vi "SerialUntraOOP.vi"(8 "error in (no error)":errorcluster, 10 "Queue In":T1) -> (0 "error out":errorcluster)   [LabVIEW 2017, in "libVariable.lvlib" / "LibFunction.lvlib"]
uses:
  LibFunction.lvlib
  <vilib>/Platform/TimedLoop/XDataNode/wakeup.ctl
  <vilib>/Platform/TimedLoop/XDataNode/XDNodeRunTimeDep.lvlib
  <vilib>/Platform/TimedLoop/XDataNode/nitl_modes.ctl
  <vilib>/Platform/TimedLoop/XDataNode/timing_clust.ctl
  <vilib>/Platform/TimedLoop/XDataNode/XDataNode.xnode
  libraryGcode/control/STATEUART.ctl
  libraryGcode/LibraryGcode.lvlib
  global/GLOBAL_STATE.vi
  libraryGcode/ClassUART/GiaoTiepUART.lvclass
  libraryGcode/control/TypeFirmwareControl.ctl
  libraryGcode/control/UartStatusBusy.ctl
  libraryGcode/control/UartCmdQueueUpdate.ctl
  libraryGcode/control/Queue/QueueCMDandPOS.ctl
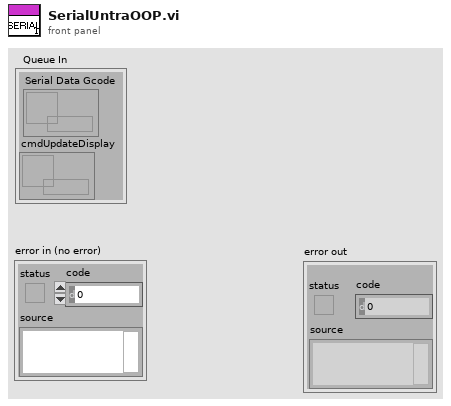
[diagram p1: front panel]
types:
  T1 = typedef "QueueCMDandPOS.ctl" = cluster{"Serial Data Gcode":refnum<queue>, "cmdUpdateDisplay":refnum<queue>}
  T2 = typedef "UartStatusBusy.ctl" = enum16{"Running", "Waiting", "Pos", "IDLE"}
  T3 = typedef "TypeFirmwareControl.ctl" = enum16{"ScaraMarlin", "CncMarlin", "Mk4Due"}
  T4 = typedef "LibraryGcode.lvlib/STATEUART.ctl" = enum16{"INIT", "WRITE", "READ", "CHECKDATA", "IDLE", "STOP"}
  T5 = typedef "XDNodeRunTimeDep.lvlib/timing_clust.ctl" = cluster{"Expected End [f-1]":u64, "Actual End [f-1]":u64, "Finished Late? [f-1]":bool, "Expected End [i-1]":u64, "Actual End [i-1]":u64, "Finished Late? [i-1]":bool, "Expected Start [i]":u64, "Actual Start [i]":u64, "Expected Start [f]":u64, "Actual Start [f]":u64, "Source Name":string, "Structure Name":string, "Period":i64, "Deadline":i64, "Offset":i64, "Start":i64, "Priority":i32, "Timeout":i32, "Mode":T6, "Wakeup Reason":T7, "Error":errorcluster, "Source Type":string, "Secondary Source Type":string, "Global End Time":u64, "Global Start Time":u64, "Frame Duration":u64, "Iteration Duration":u64, "Assigned CPU":i32, "I/O Scan Engine Mode":u32}
  T6 = typedef "XDNodeRunTimeDep.lvlib/nitl_modes.ctl" = enum32{"No Change", "Process missed periods, maintain original phase", "Discard missed periods, maintain original phase", "Process missed periods, ignore original phase", "Discard missed periods, ignore original phase"}
  T7 = typedef "XDNodeRunTimeDep.lvlib/wakeup.ctl" = enum32{"Normal", "Aborted", "Asynchronous wakeup", "Timing source error", "Timed loop error", "Timeout"}
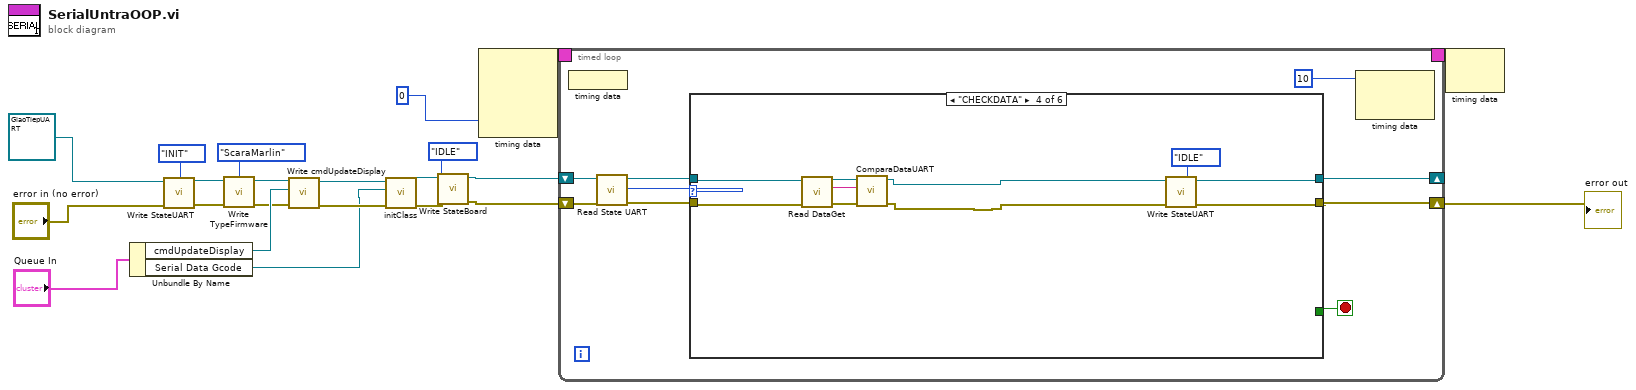
[diagram p0: block diagram]
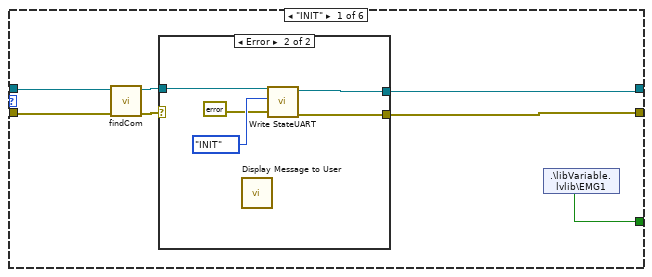
[diagram p2: hidden frame]
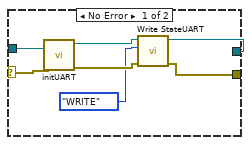
[diagram p3: hidden frame]
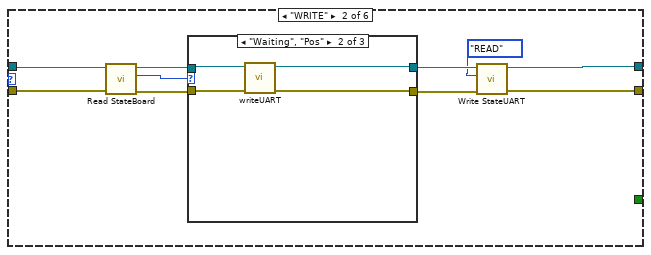
[diagram p4: hidden frame]
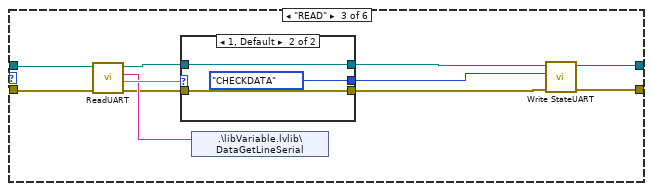
[diagram p7: hidden frame]
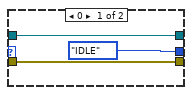
[diagram p8: hidden frame]
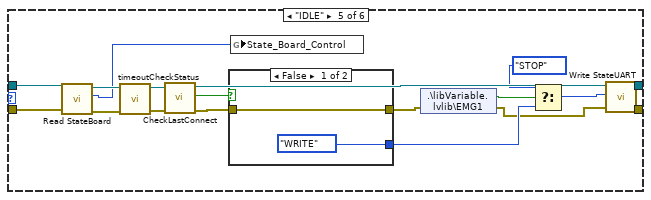
[diagram p9: hidden frame]
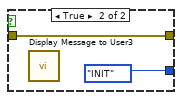
[diagram p10: hidden frame]
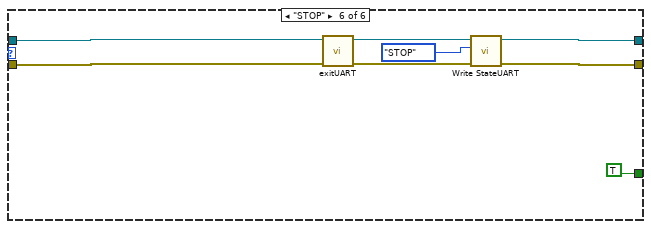
[diagram p11: hidden frame]
diagram:
  n1 = Unbundle By Name("Queue In") -> ("cmdUpdateDisplay"=w13:refnum<queue>, "Serial Data Gcode"=w6:refnum<queue>)
  n2 = call-dynamic "Write StateUART.vi"("error in (no error)"="error in (no error)", "STATEUART"=STATEUART."INIT", "GiaoTiepUART in"=refnum<class "GiaoTiepUART.lvclass"> refnum) -> ("error out"=w8:errorcluster, "GiaoTiepUART out"=w11:refnum<class "GiaoTiepUART.lvclass">)  [unwired: 7 in]
  n3 = call-dynamic "Write TypeFirmware.vi"("error in (no error)"=w8, "TypeFirmware"=TypeFirmwareControl."ScaraMarlin", "XuLyStringUART in"=w11) -> ("error out"=w9:errorcluster, "XuLyStringUART out"=w10:refnum<class "GiaoTiepUART.lvclass">)  [unwired: 7 in]
  n4 = call-dynamic "Write cmdUpdateDisplay.vi"("error in (no error)"=w9, "cmdUpdateDisplay"=w13, "XuLyStringUART in"=w10) -> ("error out"=w12:errorcluster, "XuLyStringUART out"=w15:refnum<class "GiaoTiepUART.lvclass">)  [unwired: 7 in]
  n5 = call-dynamic "initClass.vi"("error in (no error)"=w12, "Message"=w6, "GiaoTiepUART in"=w15) -> ("error out"=w2:errorcluster, "GiaoTiepUART out"=w5:refnum<class "GiaoTiepUART.lvclass">)  [unwired: 7 in]
  n6 = call-dynamic "Write StateBoard.vi"("error in (no error)"=w2, "StatePos"=UartStatusBusy."IDLE", "XuLyStringUART in"=w5) -> ("error out"=w3:errorcluster, "XuLyStringUART out"=w4:refnum<class "GiaoTiepUART.lvclass">)  [unwired: 7 in]
  n7 = node-c288(0 ("Processor")) -> (w22:T5)  [unwired: 3 in]
  n8 = timed-loop {
    timing: w22 -> [_]
    timing-out: [_] -> w21
    shift-right: [w29] -> _
    shift-left: w4 -> [w26]
    shift-right: [w28] -> w19
    shift-left: w3 -> [w27]
    stop <- w30 stop-if-true
    n9 = node-c288() -> ()  [unwired: 1 in]
    n10 = call-dynamic "Read State UART.vi"("error in (no error)"=w27, "GiaoTiepUART in"=w26) -> ("error out"=w24:errorcluster, "STATEUART"=w23:T4, "GiaoTiepUART out"=w25:refnum<class "GiaoTiepUART.lvclass">)  [unwired: 7 in]
    n11 = case shown="\"CHECKDATA\"" w23 {
      tunnel: [w34 _ _ _ _ TRUE] -> w30
      tunnel: [w38 w58 w75 w95 w108 w125] -> w29
      tunnel: w25 -> [w33 w53 w77 w92 w100 w119]
      tunnel: w24 -> [w32 w52 w76 w91 w98 w120]
      tunnel: [w35 w57 w74 w94 w107 w121] -> w28
      frame "INIT" {
        n12 = call-dynamic "findCom.vi"("error in (no error)"=w32, "GiaoTiep in"=w33) -> ("error out"=w37:errorcluster, "GiaoTiep out"=w36:refnum<class "GiaoTiepUART.lvclass">)  [unwired: 8 in]
        n13 = case shown="Error" w37 {
          selector: w37 -> [w45 _]
          tunnel: [w42 w48] -> w38
          tunnel: w36 -> [w44 w50]
          tunnel: [w43 w47] -> w35
          frame No Error {
            n14 = call-dynamic "initUART.vi"("error in (no error)"=w45, "GiaoTiep in"=w44) -> ("error out"=w40:errorcluster, "GiaoTiep out"=w41:refnum<class "GiaoTiepUART.lvclass">)  [unwired: 8 in]
            n15 = call-dynamic "Write StateUART.vi"("error in (no error)"=w40, "STATEUART"=STATEUART."WRITE", "GiaoTiepUART in"=w41) -> ("error out"=w43:errorcluster, "GiaoTiepUART out"=w42:refnum<class "GiaoTiepUART.lvclass">)  [unwired: 7 in]
          }
          frame Error {
            n16 = call "Display Message to User"() -> ()  [unwired: 10 in, 2 out]
            n17 = call-dynamic "Write StateUART.vi"("error in (no error)"=errorcluster {"status"=FALSE, "code"=30011991, "source"="NoConnect "}, "STATEUART"=STATEUART."INIT", "GiaoTiepUART in"=w50) -> ("error out"=w47:errorcluster, "GiaoTiepUART out"=w48:refnum<class "GiaoTiepUART.lvclass">)  [unwired: 7 in]
          }
        }
        n18 = shared-variable ".\\libVariable.lvlib\\EMG1"() -> (w34:bool)  [unwired: 1 in, 1 out]
      }
      frame "WRITE" {
        n19 = call-dynamic "Read StateBoard.vi"("error in (no error)"=w52, "XuLyStringUART in"=w53) -> ("error out"=w54:errorcluster, "StatePos"=w51:T2, "XuLyStringUART out"=w55:refnum<class "GiaoTiepUART.lvclass">)  [unwired: 7 in]
        n20 = case shown="\"Waiting\", \"Pos\"" w51 {
          tunnel: w55 -> [w62 w66 w68]
          tunnel: [w62 w65 w68] -> w60
          tunnel: w54 -> [w61 w64 w67]
          tunnel: [w61 w63 w67] -> w59
          frame "Running", Default {
          }
          frame "Waiting", "Pos" {
            n21 = call-dynamic "writeUART.vi"("error in (no error)"=w64, "GiaoTiep in"=w66) -> ("error out"=w63:errorcluster, "GiaoTiep out"=w65:refnum<class "GiaoTiepUART.lvclass">)  [unwired: 7 in, 1 out]
          }
          frame "IDLE" {
          }
        }
        n22 = call-dynamic "Write StateUART.vi"("error in (no error)"=w59, "STATEUART"=STATEUART."READ", "GiaoTiepUART in"=w60) -> ("error out"=w57:errorcluster, "GiaoTiepUART out"=w58:refnum<class "GiaoTiepUART.lvclass">)  [unwired: 7 in]
      }
      frame "READ" {
        n23 = call-dynamic "ReadUART.vi"("error in (no error)"=w76, "GiaoTiep in"=w77) -> ("error out"=w71:errorcluster, "milisecondGetData"=w79:dbl, "read buffer"=w78:string, "GiaoTiep out"=w70:refnum<class "GiaoTiepUART.lvclass">)  [unwired: 6 in]
        n24 = case shown="1, Default" w79 {
          tunnel: [STATEUART."IDLE" STATEUART."CHECKDATA"] -> w73
          tunnel: [w81 w84] -> w72
          tunnel: w71 -> [w81 w84]
          tunnel: [w80 w83] -> w69
          tunnel: w70 -> [w80 w83]
          frame 0 {
          }
          frame 1, Default {
          }
        }
        n25 = shared-variable ".\\libVariable.lvlib\\DataGetLineSerial"(w78) -> ()  [unwired: 1 in, 1 out]
        n26 = call-dynamic "Write StateUART.vi"("error in (no error)"=w72, "STATEUART"=w73, "GiaoTiepUART in"=w69) -> ("error out"=w74:errorcluster, "GiaoTiepUART out"=w75:refnum<class "GiaoTiepUART.lvclass">)  [unwired: 7 in]
      }
      frame "CHECKDATA" {
        n27 = call-dynamic "Read DataGet.vi"("error in (no error)"=w91, "GiaoTiepUART in"=w92) -> ("error out"=w89:errorcluster, "DataGet"=w88:string, "GiaoTiepUART out"=w90:refnum<class "GiaoTiepUART.lvclass">)  [unwired: 7 in]
        n28 = call-dynamic "ComparaDataUART.vi"("error in (no error)"=w89, "StringIN"=w88, "XuLyStringUART in"=w90) -> ("error out"=w86:errorcluster, "XuLyStringUART out"=w87:refnum<class "GiaoTiepUART.lvclass">)  [unwired: 7 in]
        n29 = call-dynamic "Write StateUART.vi"("error in (no error)"=w86, "STATEUART"=STATEUART."IDLE", "GiaoTiepUART in"=w87) -> ("error out"=w94:errorcluster, "GiaoTiepUART out"=w95:refnum<class "GiaoTiepUART.lvclass">)  [unwired: 7 in]
      }
      frame "IDLE" {
        n30 = call-dynamic "Read StateBoard.vi"("error in (no error)"=w98, "XuLyStringUART in"=w100) -> ("error out"=w97:errorcluster, "StatePos"=w96:T2, "XuLyStringUART out"=w99:refnum<class "GiaoTiepUART.lvclass">)  [unwired: 7 in]
        n31 = call-dynamic "timeoutCheckStatus.vi"("error in (no error)"=w97, "GiaoTiepUART in"=w99) -> ("error out"=w110:errorcluster, "GiaoTiepUART out"=w113:refnum<class "GiaoTiepUART.lvclass">)  [unwired: 8 in]
        n32 = call-dynamic "CheckLastConnect.vi"("error in (no error)"=w110, "GiaoTiepUART in"=w113) -> ("error out"=w102:errorcluster, "timeOut"=w112:bool, "GiaoTiepUART out"=w106:refnum<class "GiaoTiepUART.lvclass">)  [unwired: 7 in]
        n33 = case shown="False" w112 {
          tunnel: [STATEUART."WRITE" STATEUART."INIT"] -> w111
          tunnel: [w114 w116] -> w103
          tunnel: w102 -> [w114 w116]
          frame False {
          }
          frame True {
            n34 = call "Display Message to User3"() -> ()  [unwired: 10 in, 2 out]
          }
        }
        n35 = global write "GLOBAL_STATE.vi" "State_Board_Control"(w96) -> ()
        n36 = shared-variable ".\\libVariable.lvlib\\EMG1"(error in=w103) -> (w109:bool, error out=w101:errorcluster)
        n37 = Select(t=STATEUART."STOP", s=w109, f=w111) -> (s? t:f=w105:T4)
        n38 = call-dynamic "Write StateUART.vi"("error in (no error)"=w101, "STATEUART"=w105, "GiaoTiepUART in"=w106) -> ("error out"=w107:errorcluster, "GiaoTiepUART out"=w108:refnum<class "GiaoTiepUART.lvclass">)  [unwired: 7 in]
      }
      frame "STOP" {
        (unwired) TRUE
        n39 = call-dynamic "exitUART.vi"("error in (no error)"=w120, "GiaoTiep in"=w119) -> ("error out"=w122:errorcluster, "GiaoTiep out"=w123:refnum<class "GiaoTiepUART.lvclass">)  [unwired: 8 in]
        n40 = call-dynamic "Write StateUART.vi"("error in (no error)"=w122, "STATEUART"=STATEUART."STOP", "GiaoTiepUART in"=w123) -> ("error out"=w121:errorcluster, "GiaoTiepUART out"=w125:refnum<class "GiaoTiepUART.lvclass">)  [unwired: 7 in]
      }
    }
    n41 = node-c288(i64 10 ("Period")) -> ()  [unwired: 1 in, 1 out]
  }
  "error out" <- w19
  n42 = node-c288(w21) -> ()  [unwired: 1 out]
